vi "DAQmx Advance Trigger (Digital Edge).vi"(0 "task/channels in":refnum<k21>, 5 "source":tag, 7 "edge":i32(ring)=10280 items=["Rising"=10280, "Falling"=10171], 11 "error in":errorcluster) -> (4 "task out":refnum<k21>, 15 "error out":errorcluster)   [LabVIEW 2011]
doc: "Configures a switch task to advance to the next entry in a scan list on a rising or falling edge of a digital signal."
uses:
  C:/Program Files/National Instruments/LabVIEW 2011/resource/objmgr/daqmx.rc
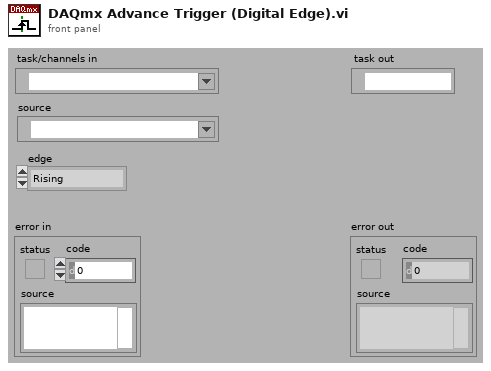
[diagram p1: front panel]
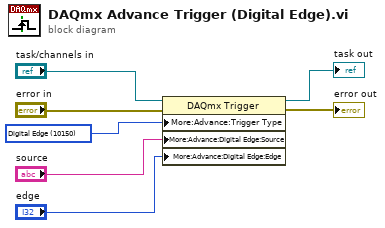
[diagram p0: block diagram]
diagram:
  w2 = 10150 items=["Digital Edge"=10150, "Software"=10292, "None"=10230] ("Advance:Trigger Type")
  n1 = property class="DAQmx Trigger"(reference="task/channels in", error in="error in", "More:Advance:Trigger Type"=w2, "More:Advance:Digital Edge:Source"="source", "More:Advance:Digital Edge:Edge"="edge") -> (reference out=→"task out":refnum<k21>, error out=→"error out":errorcluster)
